vi "generate default line.vi"(8 "error in":errorcluster, 11 "objects in":T1) -> (0 "error out":errorcluster, 2 "Line":T2, 3 "objects out":T1)   [LabVIEW 2013, in "Shared Memory editor node.lvclass"]
doc: "Generates a new line with default settings."
uses:
  Shared Memory editor node.lvclass
  module/configuration/Line.ctl
  <vilib>/NI/Tag Bus Module Framework/channel/TBM channel.lvclass
  <vilib>/NI/DCAF/Tag Editor Core/Table API/Table Manager/object ref.ctl
  <vilib>/NI/DCAF/Tag Editor Core/Configuration Editor/Classes/Engine Parent/Engine Parent Editor Node.lvclass
  <vilib>/NI/DCAF/Tag Editor Core/Configuration Editor/Classes/Module editor node/module editor node.lvclass
  <vilib>/NI/Tag Bus/tag/Data Type.ctl
  permissions.ctl
  module/configuration/Shared Memory configuration.lvclass
  <vilib>/NI/Tag Bus/tag/tag descriptor.lvclass/tag descriptor.ctl
  <vilib>/NI/Tag Bus/tag/read tag name.vi
  <vilib>/NI/Configuration Framework/serializable configuration/NISE_CEF_serializable configuration.lvclass
  <vilib>/NI/Tag Bus/tag/tag descriptor.lvclass
  <vilib>/NI/DCAF/Tag Editor Core/Table API/Table Manager/Table Manager.lvclass
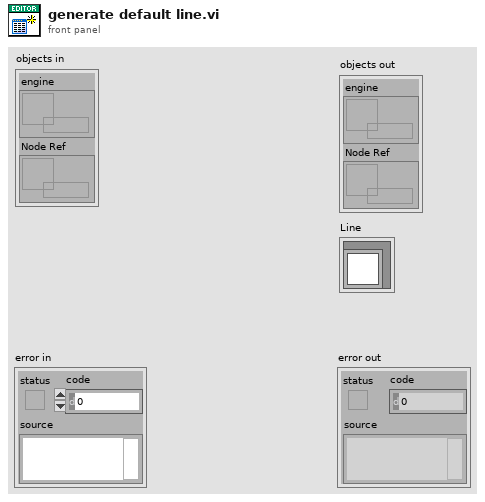
[diagram p1: front panel]
types:
  T1 = typedef "Table Manager.lvlib/Table Manager.lvclass/object ref.ctl" = cluster{"engine":refnum<data-value>, "Node Ref":refnum<data-value>}
  T2 = typedef "Shared Memory configuration.lvclass/Line.ctl" = cluster{"channel":refnum<class "TBM channel.lvclass">}
  T3 = typedef "Shared Memory editor node.lvclass/permissions.ctl" = enum32{"Read from Memory", "Write to Memory"}
  T4 = typedef "tag bus.lvlib/tag descriptor.lvclass/Data Type.ctl" = enum16{"Double", "Single", "I64", "I32", "I16", "I8", "U64", "U32", "U16", "U8", "Boolean", "String", "Array of Double", "Array of Single", "Array of I64", "Array of I32", "Array of I16", "Array of I8", "Array of U64", "Array of U32", "Array of U16", "Array of U8", "Array of Boolean", "Array of String"}
  T5 = typedef "TBM channel.lvclass/channel classification.ctl" = enum16{"input data", "output data", "processing parameter", "processing result"}
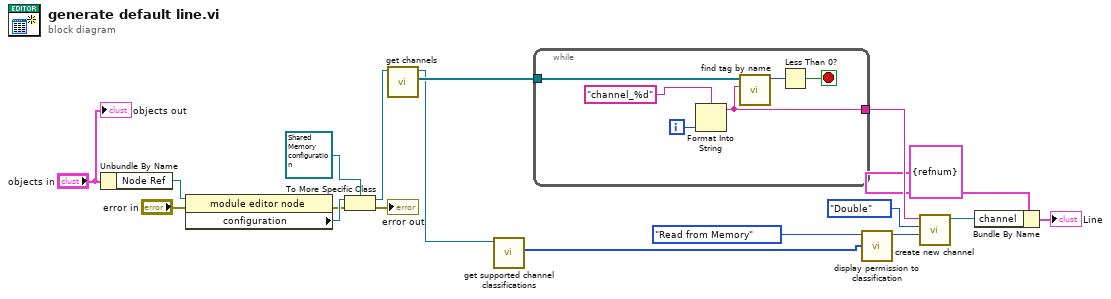
[diagram p0: block diagram]
diagram:
  n1 = Unbundle By Name("objects in") -> ("Node Ref"=w13:refnum<data-value>)
  n2 = property class="module editor node"(reference=w13, error in="error in") -> (error out=w6:errorcluster, "configuration"=w12:refnum<class "NISE_CEF_serializable configuration.lvclass">)  [unwired: 1 out]
  n3 = To More Specific Class(target class=refnum<class "Shared Memory configuration.lvclass"> refnum ("module configuration in"), reference=w12, error in=w6) -> (specific class reference=w11:refnum<class "Shared Memory configuration.lvclass">, error out=→"error out":errorcluster)
  n4 = call-dynamic "get channels.vi"("Shared Memory configuration in"=w11) -> ("channels"=w9:refnum<class "TBM channel.lvclass">[], "Shared Memory configuration out"=w2:refnum<class "Shared Memory configuration.lvclass">)  [unwired: 9 in]
  n5 = call-dynamic "get supported channel classifications.vi"("module configuration in"=w2) -> ("supported classes"=w1:T5[])  [unwired: 8 in, 2 out]
  n6 = while {
    tunnel: [w21] -> w8
    tunnel: w9 -> [w22]
    i -> [w24]
    stop <- w19 stop-if-true
    n7 = Format Into String(format string="channel_%d", w24) -> (resulting string=w21:string)  [unwired: 2 in, 1 out]
    n8 = call <vilib>:"find tag by name.vi"("name"=w21, "tags in"=w22) -> ("index"=w20:i32)  [unwired: 9 in]
    n9 = Less Than 0?(x=w20) -> (x < 0?=w19:bool)
  }
  n10 = call "display permission to classification.vi"("supported classes"=w1, "display permissions"=permissions."Read from Memory") -> ("channel classification"=w14:T5)  [unwired: 9 in]
  n11 = call <vilib>:"create new channel.vi"("channel classification"=w14, "data type"=Data_Type."Double", "channel name"=w8) -> ("channel"=w17:refnum<class "TBM channel.lvclass">)  [unwired: 8 in]
  n12 = Bundle By Name(cluster=T2 {"channel"=refnum} ("Line"), "channel"=w17) -> (→"Line":T2)
  "objects out" <- "objects in"
